vi "Create If File Does Not Exist.vi"(8 "error in (no error)":errorcluster, 11 "User Preferences File in":refnum<class "User Preferences File.lvclass">) -> (0 "error out":errorcluster, 3 "User Preferences File out":refnum<class "User Preferences File.lvclass">)   [LabVIEW 2020, in "RxnRover.lvlib" / "User Preferences File.lvclass"]
doc: "Creates the user preferences file with default values if it does not exist. The Init VI or custom values for file name and location must be set before running this VI."
uses:
  User Preferences File.lvclass
  User Preferences File.lvclass/User Preferences File.ctl
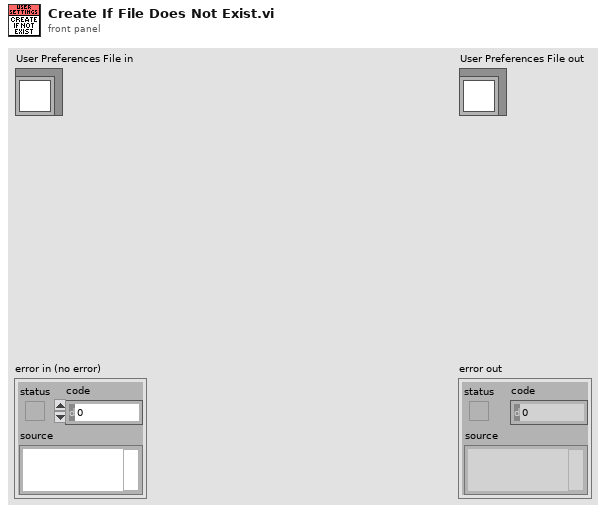
[diagram p1: front panel]
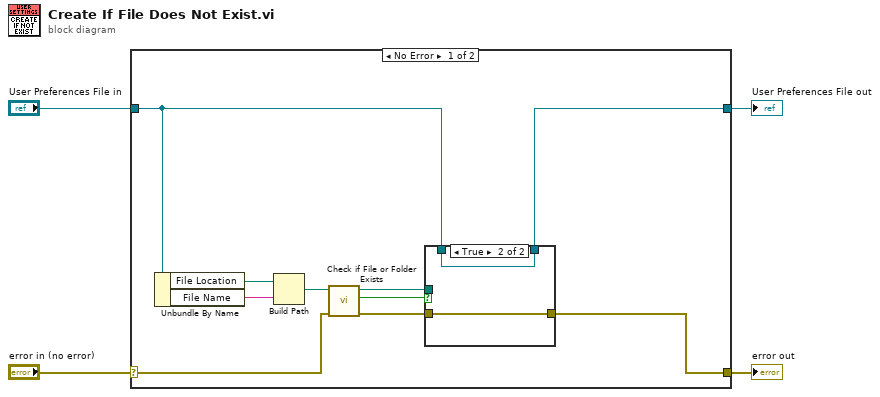
[diagram p0: block diagram]
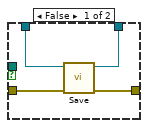
[diagram p2: hidden frame]
diagram:
  n1 = case shown="No Error" "error in (no error)" {
    selector: "error in (no error)" -> [w10 w22]
    tunnel: [w12 w22] -> w3
    tunnel: [w5 w21] -> w1
    tunnel: "User Preferences File in" -> [w6 w21]
    frame No Error {
      n2 = Unbundle By Name(w6) -> ("File Location"=w14:path, "File Name"=w13:string)
      n3 = Build Path(base path=w14, name or relative path=w13) -> (appended path=w11:path)
      n4 = call <vilib>:"Check if File or Folder Exists.vi"("error in (no error)"=w10, "path"=w11) -> ("error out"=w7:errorcluster, "file or folder exists?"=w9:bool, "dup path"=w8:path)  [unwired: 7 in]
      n5 = case shown="True" w9 {
        tunnel: [w17 w20] -> w12
        tunnel: w8 -> [_ _]
        tunnel: w7 -> [w18 w20]
        tunnel: w6 -> [w16 w19]
        tunnel: [w15 w19] -> w5
        frame False {
          n6 = call "Save.vi"("error in (no error)"=w18, "User Preferences File in"=w16) -> ("error out"=w17:errorcluster, "User Preferences File out"=w15:refnum<class "User Preferences File.lvclass">)  [unwired: 8 in]
        }
        frame True {
        }
      }
    }
    frame Error {
    }
  }
  "error out" <- w3
  "User Preferences File out" <- w1
